vi "Create Actual Table Name.vi"(11 "Name or Path":string) -> (3 "Absolute Path":string)   [LabVIEW 2017]
doc: "If input is a relative path, turn it into an absolute SmartDashboard path."
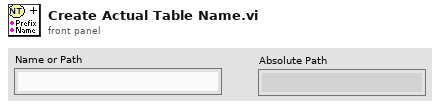
[diagram p1: front panel]
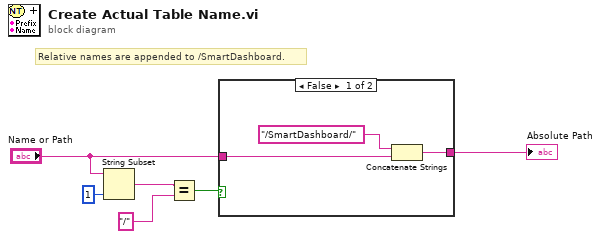
[diagram p0: block diagram]
diagram:
  # "Relative names are appended to /SmartDashboard."
  n1 = String Subset(string="Name or Path", length (rest)=1 ("length (rest)")) -> (substring=w1:string)  [unwired: 1 in]
  n2 = Equal?(x=w1, y="/") -> (x = y?=w3:bool)
  n3 = case shown="False" w3 {
    tunnel: "Name or Path" -> [w8 w10]
    tunnel: [w9 w10] -> w4
    frame False {
      n4 = Concatenate Strings("/SmartDashboard/", w8) -> (w9:string)
    }
    frame True {
    }
  }
  "Absolute Path" <- w4
